vi "getScriptEvent.vi"(8 "error in (no error)":errorcluster, 11 "ActionPanel.lvclass in":refnum<class "ActionPanel.lvclass">) -> (0 "error out":errorcluster, 2 "ScriptEvent.lvclass":refnum<class "ScriptEvent.lvclass">, 3 "ActionPanel.lvclass out":refnum<class "ActionPanel.lvclass">)   [LabVIEW 2009, in "Views.lvlib" / "ScriptEditor.lvlib" / "ActionPanel.lvclass"]
uses:
  ActionPanel.lvclass
  Tools/Scripting/ScriptingEvent/ScriptEvent.lvclass
  ActionPanel.lvclass/ActionPanel.ctl
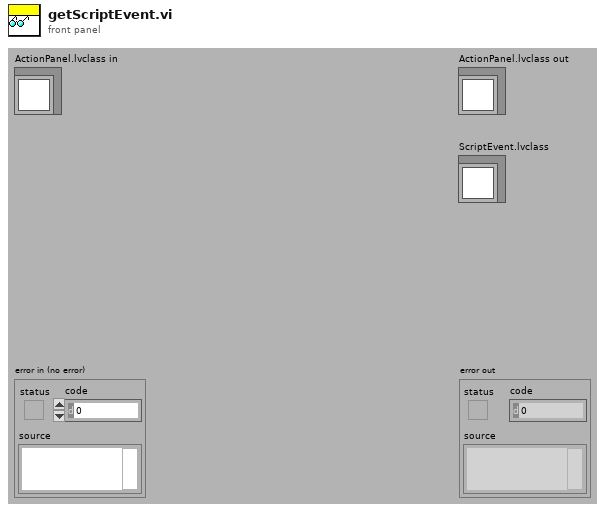
[diagram p1: front panel]
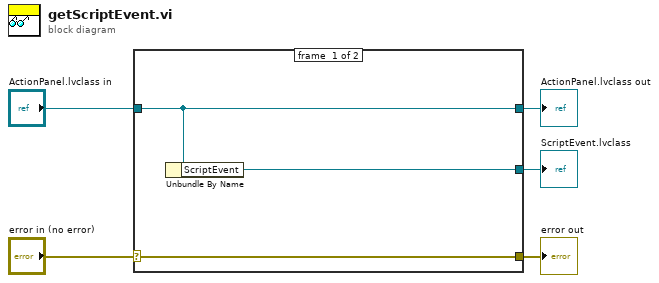
[diagram p0: block diagram]
diagram:
  n1 = case shown="No Error" "error in (no error)" {
    selector: "error in (no error)" -> [w8 w9]
    tunnel: [w8 w9] -> w4
    tunnel: [w7 w10] -> w2
    tunnel: "ActionPanel.lvclass in" -> [w7 w10]
    tunnel: [w6 _] -> w1
    frame #0 {
      n2 = Unbundle By Name(w7) -> ("ScriptEvent"=w6:refnum<class "ScriptEvent.lvclass">)
    }
    frame #1 {
    }
  }
  "error out" <- w4
  "ActionPanel.lvclass out" <- w2
  "ScriptEvent.lvclass" <- w1
